vi "Register and Process SAL events.vi"(8 "error in (no error)":errorcluster, 9 "M1M3 Support Events in":refnum<class "M1M3 Support Events.lvclass">, 10 "User Events in":refnum<class "User Events.lvclass">, 11 "Boot Loader in":refnum<class "Boot Loader.lvclass">) -> (0 "error out":errorcluster, 3 "Boot Loader out":refnum<class "Boot Loader.lvclass">)   [LabVIEW 2016, in "Boot Loader.lvclass"]
uses:
  Boot Loader.lvclass
  User Events/User Events.lvclass
  M1M3 Support Events/M1M3 Support Events.lvclass
  User Events/User Events.lvclass/User Events.ctl
  Typedefs/StateTypes.ctl
  SALLV_m1m3/SALLV_m1m3.lvlib
  Typedefs/M1M3SupportEUI_TypeDefs.lvlib
panel:
  out "Boolean":bool
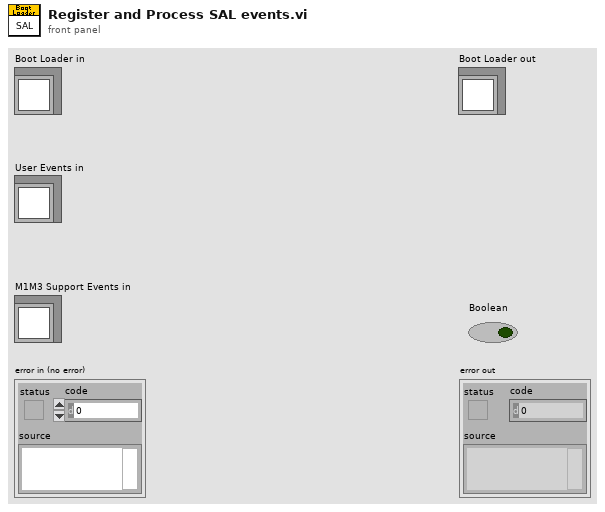
[diagram p1: front panel]
types:
  T1 = typedef "M1M3SupportEUI_TypeDefs.lvlib/Publish Data Events.ctl" = cluster{"State":refnum<user-event>, "ErrorCode":refnum<user-event>}
  T2 = typedef "M1M3SupportEUI_TypeDefs.lvlib/StateTypes.ctl" = enum16{"Offline State", "Fault State", "Standby State", "Disabled State", "Enabled State", "Wait For User Input State", "Test Actuator State"}
  T3 = typedef "SALLV_m1m3.lvlib/logevent_SummaryState.ctl" = cluster{"Timestamp":dbl, "SummaryState":i32, "priority":i32}
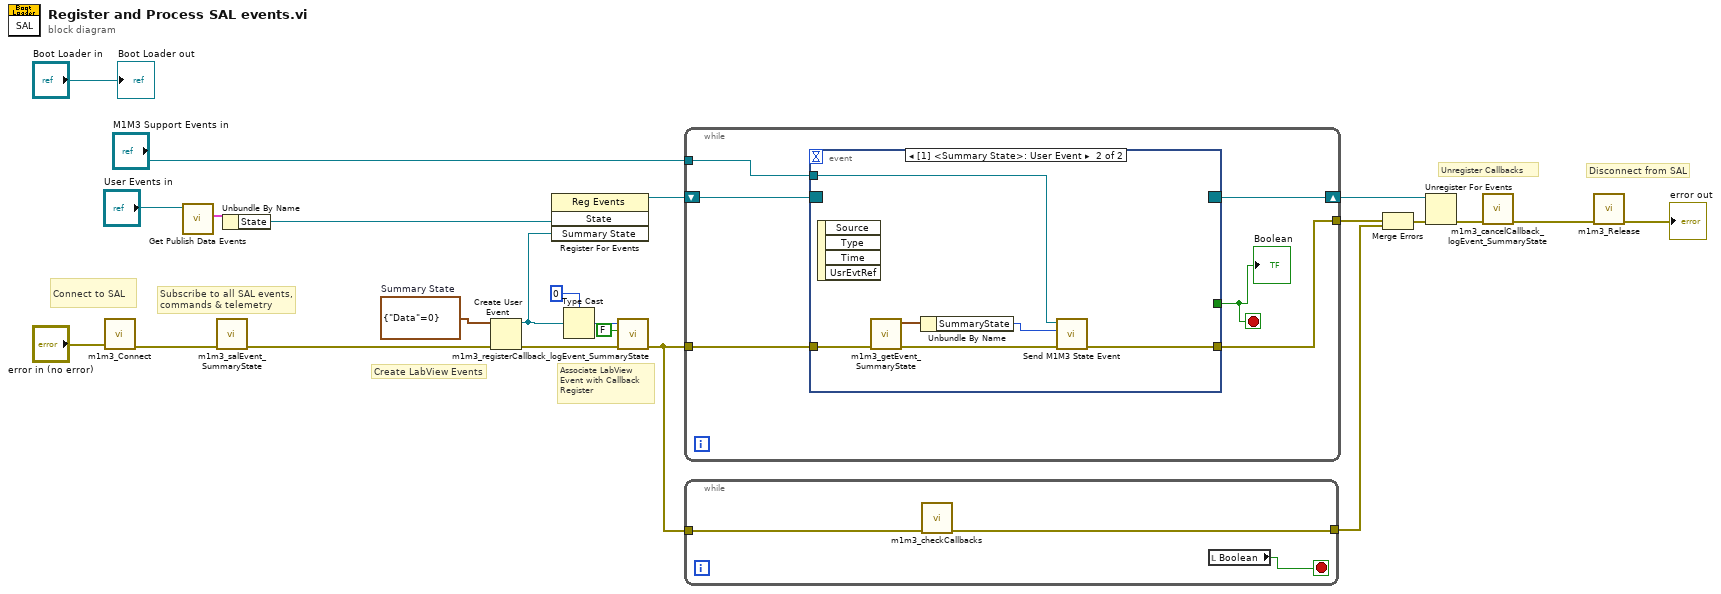
[diagram p0: block diagram]
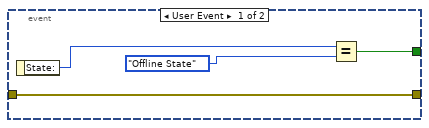
[diagram p2: hidden frame]
diagram:
  w12 = cluster{"Data":i32} {"Data"=0}  # Summary State
  # "Associate LabView\nEvent with Callback\nRegister"
  # "Create LabView Events"
  # "Disconnect from SAL"
  # "Unregister Callbacks"
  # "Subscribe to all SAL events, \ncommands & telemetry"
  # "Connect to SAL"
  n1 = call "m1m3_Connect.vi"("error in (no error)"="error in (no error)") -> ("error out"=w15:errorcluster)  [unwired: 9 in, 1 out]
  n2 = call "Get Publish Data Events.vi"("UserEvents in"="User Events in") -> ("Publish Data Events"=w20:T1)  [unwired: 9 in, 1 out]
  n3 = call "m1m3_salEvent_SummaryState.vi"("error in (no error)"=w15) -> ("error out"=w11:errorcluster)  [unwired: 9 in, 1 out]
  n4 = Unbundle By Name(w20) -> ("State"=w19:refnum<user-event>)
  n5 = Create User Event(user event datatype=w12, error in=w11) -> (user event=w10:refnum<user-event>, error out=w7:errorcluster)
  n6 = register-events(w19, w10) -> (reference out=w18:refnum<event-registration>)  [unwired: 2 in, 1 out]
  n7 = Type Cast(type=0, x=w10) -> (*(type *) &x=w8:i32)
  n8 = call "m1m3_registerCallback_logEvent_SummaryState.vi"("error in (no error)"=w7, "skipOld"=FALSE, "handle"=w8) -> ("error out"=w4:errorcluster)  [unwired: 7 in, 1 out]
  n9 = while {
    shift-right: [w28] -> w17
    shift-left: w18 -> [w29]
    tunnel: w4 -> [w27]
    tunnel: "M1M3 Support Events in" -> [w26]
    tunnel: [w25] -> w2
    stop <- w24 stop-if-true
    n10 = event shown="[1] <Summary State>: User Event" {
      selector: w29 -> [_ _]
      dyn-events: [_ _] -> w28
      timeout: _ -> [_ _]
      tunnel: [w31 _] -> w24
      tunnel: w27 -> [w30 w39]
      tunnel: w26 -> [_ w38]
      tunnel: [w30 w34] -> w25
      event User Event {
        n11 = event-data() -> ("State:"=w32:T2)  [unwired: 1 in]
        n12 = Equal?(x=w32, y=StateTypes."Offline State") -> (x = y?=w31:bool)
      }
      event User Event {
        n13 = event-data() -> ()  [unwired: 1 in, 4 out]
        n14 = call "m1m3_getEvent_SummaryState.vi"("error in (no error)"=w39) -> ("error out"=w35:errorcluster, "logevent_SummaryState_Ctl out"=w37:T3)  [unwired: 8 in, 1 out]
        n15 = Unbundle By Name(w37) -> ("SummaryState"=w36:i32)
        n16 = call "Send M1M3 State Event.vi"("error in (no error)"=w35, "M1M3 Support State"=w36, "M1M3 Support Events in"=w38) -> ("error out"=w34:errorcluster)  [unwired: 7 in, 1 out]
      }
    }
    "Boolean" <- w24
  }
  n17 = while {
    tunnel: w4 -> [w41]
    tunnel: [w40] -> w1
    stop <- w42 stop-if-true
    n18 = call "m1m3_checkCallbacks.vi"("error in (no error)"=w41) -> ("error out"=w40:errorcluster)  [unwired: 10 in]
    n19 = local read "Boolean"() -> (w42:bool)
  }
  n20 = Merge Errors(w2, w1) -> (w3:errorcluster)
  n21 = Unregister For Events(event registration refnum=w17, error in=w3) -> (error out=w14:errorcluster)
  n22 = call "m1m3_cancelCallback_logEvent_SummaryState.vi"("error in (no error)"=w14) -> ("error out"=w13:errorcluster)  [unwired: 9 in, 1 out]
  n23 = call "m1m3_Release.vi"("error in (no error)"=w13) -> ("error out"=→"error out":errorcluster)  [unwired: 9 in, 1 out]
  "Boot Loader out" <- "Boot Loader in"
